vi "ShiftStoneColor.vi"(7 "StoneColor in":u16) -> (8 "StoneColor out":u16)   [LabVIEW 2009]
doc: "Change the stone color. White to Black/Black to white."
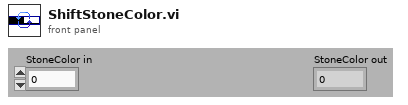
[diagram p1: front panel]
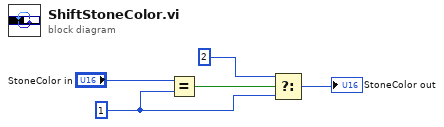
[diagram p0: block diagram]
diagram:
  w2 = u16 1 ("y")
  n1 = Equal?(x="StoneColor in", y=w2) -> (x = y?=w4:bool)
  n2 = Select(t=u16 2 ("y"), s=w4, f=w2) -> (s? t:f=→"StoneColor out":u16)
